vi "PM_DateTime_DEMO.vi"() -> (0 "error out":errorcluster, 1 "TIEMPO_MEDICION":string)   [LabVIEW 2018]
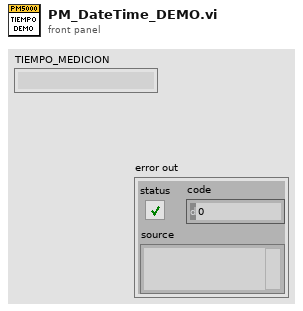
[diagram p1: front panel]
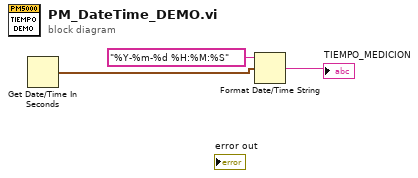
[diagram p0: block diagram]
diagram:
  n1 = Get Date/Time In Seconds() -> (seconds since 1Jan1904=w1:timestamp)
  n2 = Format Date/Time String(time format string (%c)="%Y-%m-%d %H:%M:%S", seconds (now)=w1) -> (date/time string=→"TIEMPO_MEDICION":string)  [unwired: 1 in]
